vi "Split TargetPanel by Node.vi"(6 "Dynamic VI*":refnum<vi>, 8 "error in":errorcluster caption="错误输入（无错误）", 9 "Split Mode":T1, 10 "Node*":refnum<data-value>, 11 "PanelRootNode 输入":refnum<class "PanelRootNode.lvclass"> caption="DNL_LabVIEW Object in") -> (0 "error out":errorcluster caption="错误输出", 2 "ChildDataNode[]":refnum<data-value>[](array[refnum]), 3 "PanelRootNode 输出":refnum<class "PanelRootNode.lvclass"> caption="DNL_LabVIEW Object out")   [LabVIEW 2016, in "PanelRootNode.lvclass"]
uses:
  PanelRootNode.lvclass
  C:/Users/CL/Desktop/ZcDAQprj0811/ZcDAQprj/Modules/DAQ-Display/PanelSplitToolkit/PanelLinkNode/PanelLinkNode.lvclass
  PanelObject/PanelObject.lvclass
  PanelDataNode/Split Mode.ctl
  PanelDataNode/PanelDataNode.lvclass
  C:/Users/CL/Desktop/ZcDAQprj0811/ZcDAQprj/Modules/DAQ-Display/PanelSplitToolkit/PanelObject/PanelObject.lvclass
  PanelLinkNode/PanelLinkNode.lvclass/PanelLinkNode.ctl
  PanelLinkNode/PanelLinkNode.lvclass
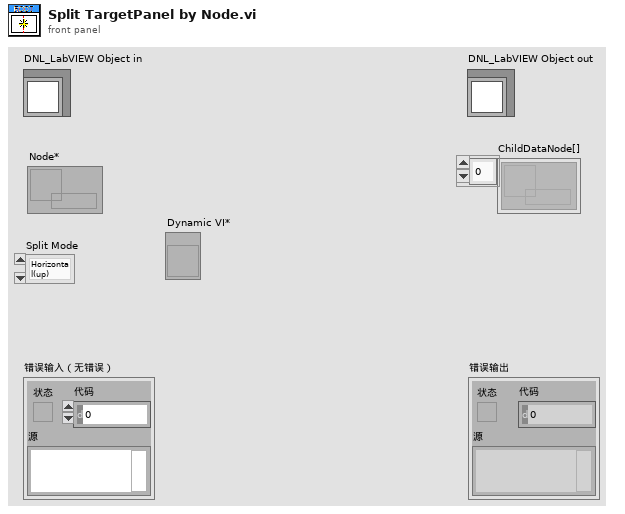
[diagram p1: front panel]
types:
  T1 = typedef "PanelDataNode.lvclass/Split Mode.ctl" = enum16{"Horizontal(up)", "Vertical(left)", "Horizontal(down)", "Vertical(right)"}
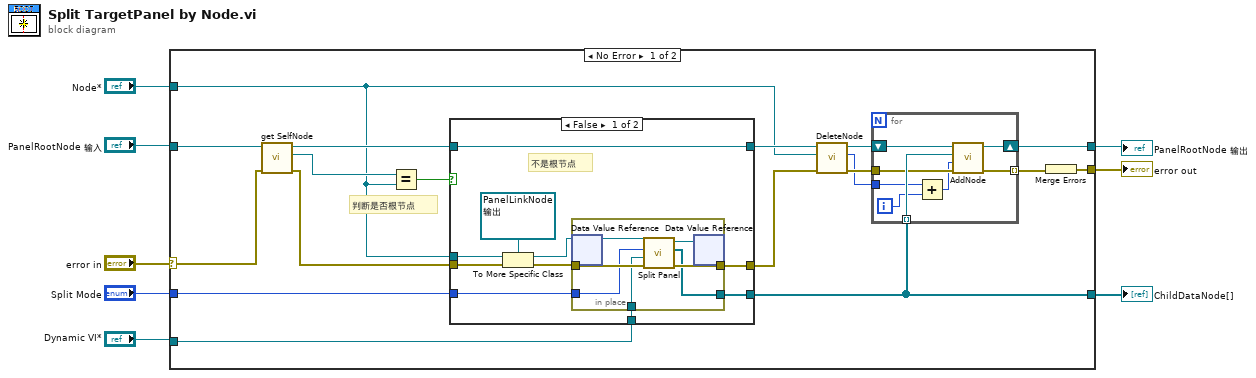
[diagram p0: block diagram]
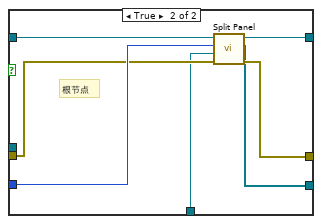
[diagram p2: hidden frame]
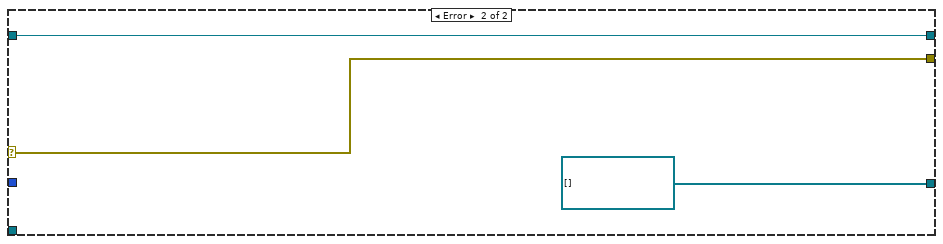
[diagram p3: hidden frame]
diagram:
  n1 = case shown="No Error" "error in" {
    selector: "error in" -> [w18 w61]
    tunnel: [w11 w61] -> w4
    tunnel: [w15 w60] -> w8
    tunnel: "PanelRootNode 输入" -> [w22 w60]
    tunnel: "Node*" -> [w17 _]
    tunnel: "Split Mode" -> [w23 _]
    tunnel: [w14 refnum<data-value>[] [] ("ChildDataNode[]")] -> w2
    tunnel: "Dynamic VI*" -> [w9 _]
    frame No Error {
      # "判断是否根节点"
      n2 = call "get SelfNode.vi"("error in (no error)"=w18, "PanelLinkNode输入"=w22) -> ("error out"=w19:errorcluster, "SelfNode*"=w25:refnum<data-value>, "PanelLinkNode输出"=w26:refnum<class "PanelRootNode.lvclass">)  [unwired: 7 in]
      n3 = Equal?(x=w25, y=w17) -> (x = y?=w24:bool)
      n4 = case shown="False" w24 {
        tunnel: [w44 w58] -> w20
        tunnel: w26 -> [w43 w57]
        tunnel: [w43 w56] -> w21
        tunnel: w17 -> [w40 _]
        tunnel: w23 -> [w38 w55]
        tunnel: [w37 w54] -> w14
        tunnel: w19 -> [w36 w53]
        tunnel: w9 -> [w35 w52]
        frame False {
          # "不是根节点"
          n5 = To More Specific Class(target class=refnum<data-value> refnum ("数据值引用"), reference=w40, error in=w36) -> (specific class reference=w42:refnum<data-value>, error out=w41:errorcluster)
          n6 = in-place {
            in-place-border: w41 -> [w48]
            in-place-border: [w49] -> w44
            in-place-border: w38 -> [w47]
            in-place-border: [w46] -> w37
            in-place-border: w35 -> [w45]
            n7 = in-place-dvr #1(w42) -> (w51:refnum<class "PanelRootNode.lvclass">)  [unwired: 1 out]
            n8 = call-dynamic "Split Panel.vi"("error in"=w48, "VI*"=w45, "Split Mode"=w47, "PanelDataNode 输入"=w51) -> ("error out"=w49:errorcluster, "ChildDataNode[]"=w46:refnum<data-value>[], "PanelDataNode 输出"=w50:refnum<class "PanelRootNode.lvclass">)  [unwired: 5 in]
            n9 = in-place-dvr #1(w50) -> ()  [unwired: 2 out]
          }
        }
        frame True {
          # "根节点"
          n10 = call-dynamic "Split Panel.vi"("error in"=w53, "VI*"=w52, "Split Mode"=w55, "PanelDataNode 输入"=w57) -> ("error out"=w58:errorcluster, "ChildDataNode[]"=w54:refnum<data-value>[], "PanelDataNode 输出"=w56:refnum<class "PanelRootNode.lvclass">)  [unwired: 5 in]
        }
      }
      n11 = call "DeleteNode.vi"("error in (no error)"=w20, "Node*"=w17, "PanelRootNode 输入"=w21) -> ("error out"=w13:errorcluster, "index"=w10:i32, "PanelRootNode 输出"=w16:refnum<class "PanelRootNode.lvclass">)  [unwired: 6 in]
      n12 = for {
        tunnel: w14 -> [w32] mode=indexing
        tunnel: w13 -> [w31]
        shift-right: [w33] -> w15
        shift-left: w16 -> [w34]
        tunnel: [w30] -> w12 mode=indexing
        tunnel: w10 -> [w29]
        i -> [w28]
        n13 = Add(x=w29, y=w28) -> (x+y=w27:i32)
        n14 = call "AddNode.vi"("error in (no error)"=w31, "Index"=w27, "Node*"=w32, "PanelRootNode 输入"=w34) -> ("error out"=w30:errorcluster, "PanelRootNode 输出"=w33:refnum<class "PanelRootNode.lvclass">)  [unwired: 6 in]
      }
      n15 = Merge Errors(w12) -> (w11:errorcluster)
    }
    frame Error {
    }
  }
  "error out" <- w4
  "PanelRootNode 输出" <- w8
  "ChildDataNode[]" <- w2
